vi "SYST_UPR_LOAD.vi"(0 "VISA IN":refnum<visa-resource-name>, 5 "error in":errorcluster, 7 "FileName":string) -> (14 "VISA Out":refnum<visa-resource-name>, 19 "error out":errorcluster)   [LabVIEW 2018, in "PNA-X.lvlib"]
doc: "SYSTem:UPReset:LOAD <file> \n(Read-Write) Loads an existing instrument state file (.sta or .cst) to be used for User Preset. \nSubsequent execution of SYSTem:UPReset will cause the PNA to assume this instrument state. \nRegardless of the state of the User Preset Enable checkbox, the SYST:PRESet command will always \npreset the PNA to the factory preset settings, and SYST:UPReset will always perform a User Preset. \nLearn more about User Preset. \nParameters \n<file> String - Name of the file to be loaded. The default folder \"C:\\Program \nFiles\\Agilent\\Network Analyzer\\Documents\" is used if unspecified. Change \nthe default folder name using MMEMory:CDIRectory. \nExamples SYST:UPR:LOAD '1MHzto20GHzUserPreset.cst' \nsystem:upreset:load 'C:\\Documents and Settings\\Administrator\\My \nDocuments\\NewUserPreset.cst' \nQuery Syntax Not Applicable \nDefault Not Applicable"
uses:
  PNA-X.lvlib
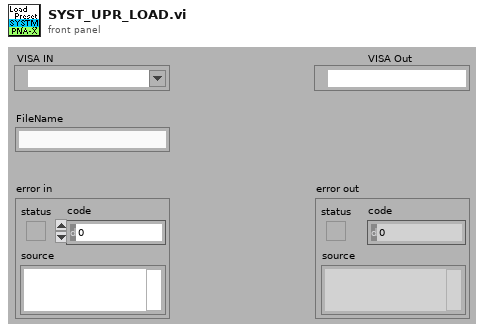
[diagram p1: front panel]
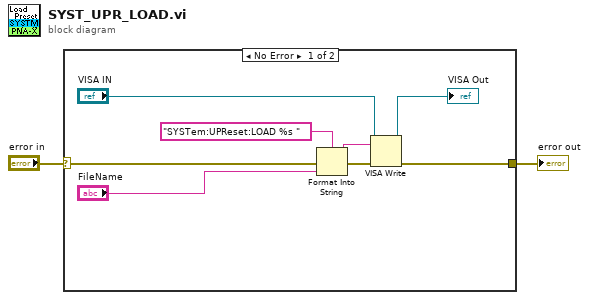
[diagram p0: block diagram]
diagram:
  n1 = case shown="No Error" "error in" {
    selector: "error in" -> [w10 w11]
    tunnel: [w5 w11] -> w1
    frame No Error {
      n2 = Format Into String(format string="SYSTem:UPReset:LOAD %s " ("Cmdline"), error in=w10, "FileName") -> (resulting string=w8:string, error out=w9:errorcluster)  [unwired: 1 in]
      n3 = VISA Write(VISA resource name="VISA IN", write buffer=w8, error in (no error)=w9) -> (VISA resource name out=→"VISA Out":refnum<visa-resource-name>, error out=w5:errorcluster)  [unwired: 1 out]
    }
    frame Error {
    }
  }
  "error out" <- w1
